vi "Preset PART NUMBER.vi"(1 "PART number":string, 8 "error in (no error)":errorcluster, 11 "VISA resource in":refnum<visa-resource-name>) -> (0 "error out":errorcluster, 3 "VISA resource out":refnum<visa-resource-name>)   [LabVIEW 2025]
uses:
  serial__lot_part_number_states.ctl
  <instrlib>/Chroma 19052/Chroma 19052.lvlib
panel:
  # "Min 1 char, Max 13 char"
  # "Set PART number"
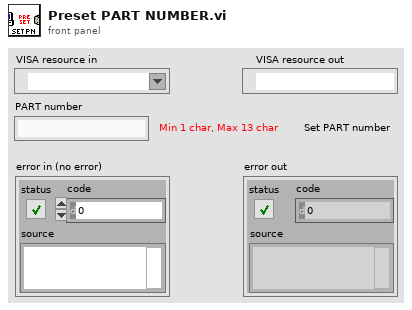
[diagram p1: front panel]
types:
  T1 = typedef "serial__lot_part_number_states.ctl" = enum16{"Initialize", "check <=UL", "check >=LL", "trim", "write", "Shutdown"}
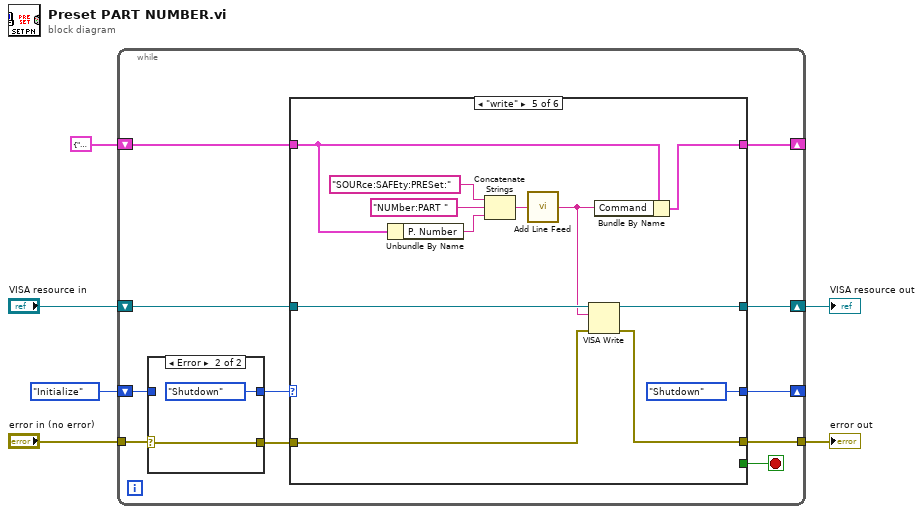
[diagram p0: block diagram]
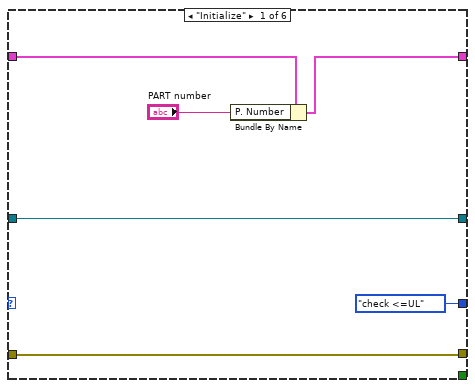
[diagram p3: hidden frame]
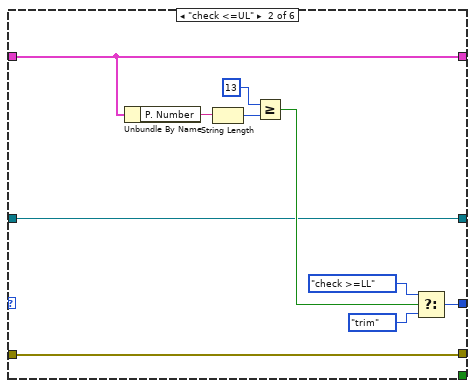
[diagram p4: hidden frame]
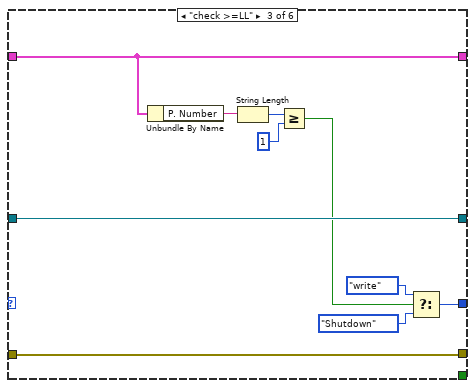
[diagram p5: hidden frame]
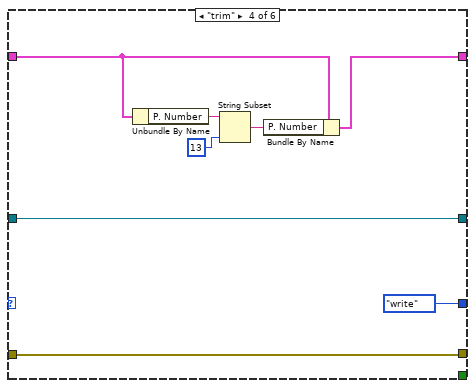
[diagram p6: hidden frame]
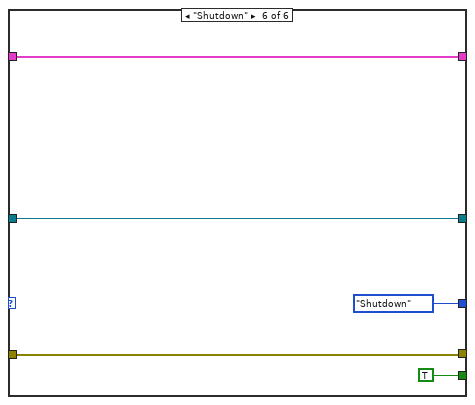
[diagram p7: hidden frame]
diagram:
  n1 = while {
    tunnel: "error in (no error)" -> [w16]
    shift-right: [w15] -> _
    shift-left: serial__lot_part_number_states."Initialize" -> [w14]
    tunnel: [w11] -> w4
    shift-right: [w10] -> w3
    shift-left: "VISA resource in" -> [w13]
    shift-right: [w8] -> _
    shift-left: cluster{"P. Number":string, "Command":string} {"P. Number"="", "Command"=""} -> [w7]
    stop <- w9 stop-if-true
    n2 = case shown="Error" w16 {
      selector: w16 -> [w19 w20]
      tunnel: [w19 w20] -> w12
      tunnel: [w18 serial__lot_part_number_states."Shutdown"] -> w17
      tunnel: w14 -> [w18 _]
      frame No Error {
      }
      frame Error {
      }
    }
    n3 = case shown="\"write\"" w17 {
      tunnel: [serial__lot_part_number_states."check <=UL" w34 w43 serial__lot_part_number_states."write" serial__lot_part_number_states."Shutdown" serial__lot_part_number_states."Shutdown"] -> w15
      tunnel: w13 -> [w26 w32 w47 w55 w67 w72]
      tunnel: w12 -> [w27 w31 w46 w54 w66 w71]
      tunnel: [w27 w31 w46 w54 w65 w71] -> w11
      tunnel: [w26 w32 w47 w55 w64 w72] -> w10
      tunnel: [_ _ _ _ _ TRUE] -> w9
      tunnel: w7 -> [w24 w29 w39 w49 w58 w68]
      tunnel: [w23 w29 w39 w48 w56 w68] -> w8
      frame "Initialize" {
        n4 = Bundle By Name(cluster=w24, "P. Number"="PART number") -> (w23:cluster{"P. Number":string, "Command":string})
      }
      frame "check <=UL" {
        n5 = Unbundle By Name(w29) -> ("P. Number"=w28:string)
        n6 = String Length(string=w28) -> (length=w36:i32)
        n7 = Greater Or Equal?(x=13 ("y"), y=w36) -> (x >= y?=w35:bool)
        n8 = Select(t=serial__lot_part_number_states."check >=LL", s=w35, f=serial__lot_part_number_states."trim") -> (s? t:f=w34:T1)
      }
      frame "check >=LL" {
        n9 = Unbundle By Name(w39) -> ("P. Number"=w38:string)
        n10 = String Length(string=w38) -> (length=w45:i32)
        n11 = Greater Or Equal?(x=w45, y=1) -> (x >= y?=w41:bool)
        n12 = Select(t=serial__lot_part_number_states."write", s=w41, f=serial__lot_part_number_states."Shutdown") -> (s? t:f=w43:T1)
      }
      frame "trim" {
        n13 = Unbundle By Name(w49) -> ("P. Number"=w51:string)
        n14 = String Subset(string=w51, length (rest)=13 ("length (rest)")) -> (substring=w50:string)  [unwired: 1 in]
        n15 = Bundle By Name(cluster=w49, "P. Number"=w50) -> (w48:cluster{"P. Number":string, "Command":string})
      }
      frame "write" {
        n16 = Unbundle By Name(w58) -> ("P. Number"=w60:string)
        n17 = Concatenate Strings("SOURce:SAFEty:PRESet:", "NUMber:PART ", w60) -> (w59:string)
        n18 = call <instrlib>:"Add Line Feed.vi"("Command string"=w59) -> ("Concatenated string"=w57:string)  [unwired: 4 in]
        n19 = VISA Write(VISA resource name=w67, write buffer=w57, error in (no error)=w66) -> (VISA resource name out=w64:refnum<visa-resource-name>, error out=w65:errorcluster)  [unwired: 1 out]
        n20 = Bundle By Name(cluster=w58, "Command"=w57) -> (w56:cluster{"P. Number":string, "Command":string})
      }
      frame "Shutdown" {
      }
    }
  }
  "error out" <- w4
  "VISA resource out" <- w3
